vi "160041036.vi"() -> ()   [LabVIEW 2018]
panel:
  out "CAR":bool
  out "Boolean 19":bool
  out "Boolean 18":bool
  out "Boolean 17":bool
  out "Boolean 16":bool
  out "Boolean 15":bool
  out "Boolean 14":bool
  out "?":bool
  out "?":bool
  out "Boolean 13":bool
  out "Boolean 12":bool
  out "?":bool
  out "car 4":bool
  out "car 3":bool
  out "car2":bool
  out "1":bool
  out "2":bool
  in  "Boolean 11":bool
  in  "Boolean 10":bool
  in  "Boolean 9":bool
  in  "Boolean 8":bool
  in  "Boolean 7":bool
  in  "Boolean 6":bool
  in  "Boolean 5":bool
  in  "Boolean 4":bool
  in  "Boolean 3":bool
  in  "Boolean 2":bool
  in  "Boolean":bool
  # "R.R. MALL PARKING"
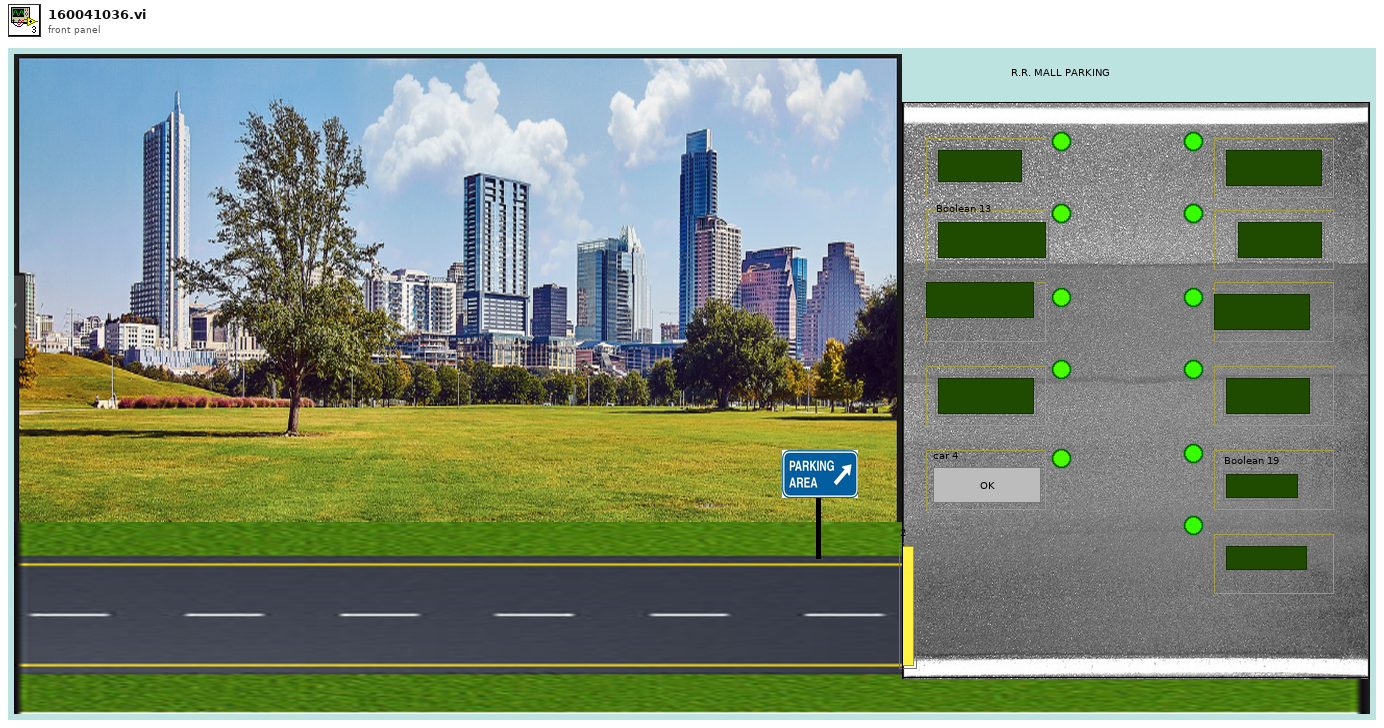
[diagram p1: front panel]
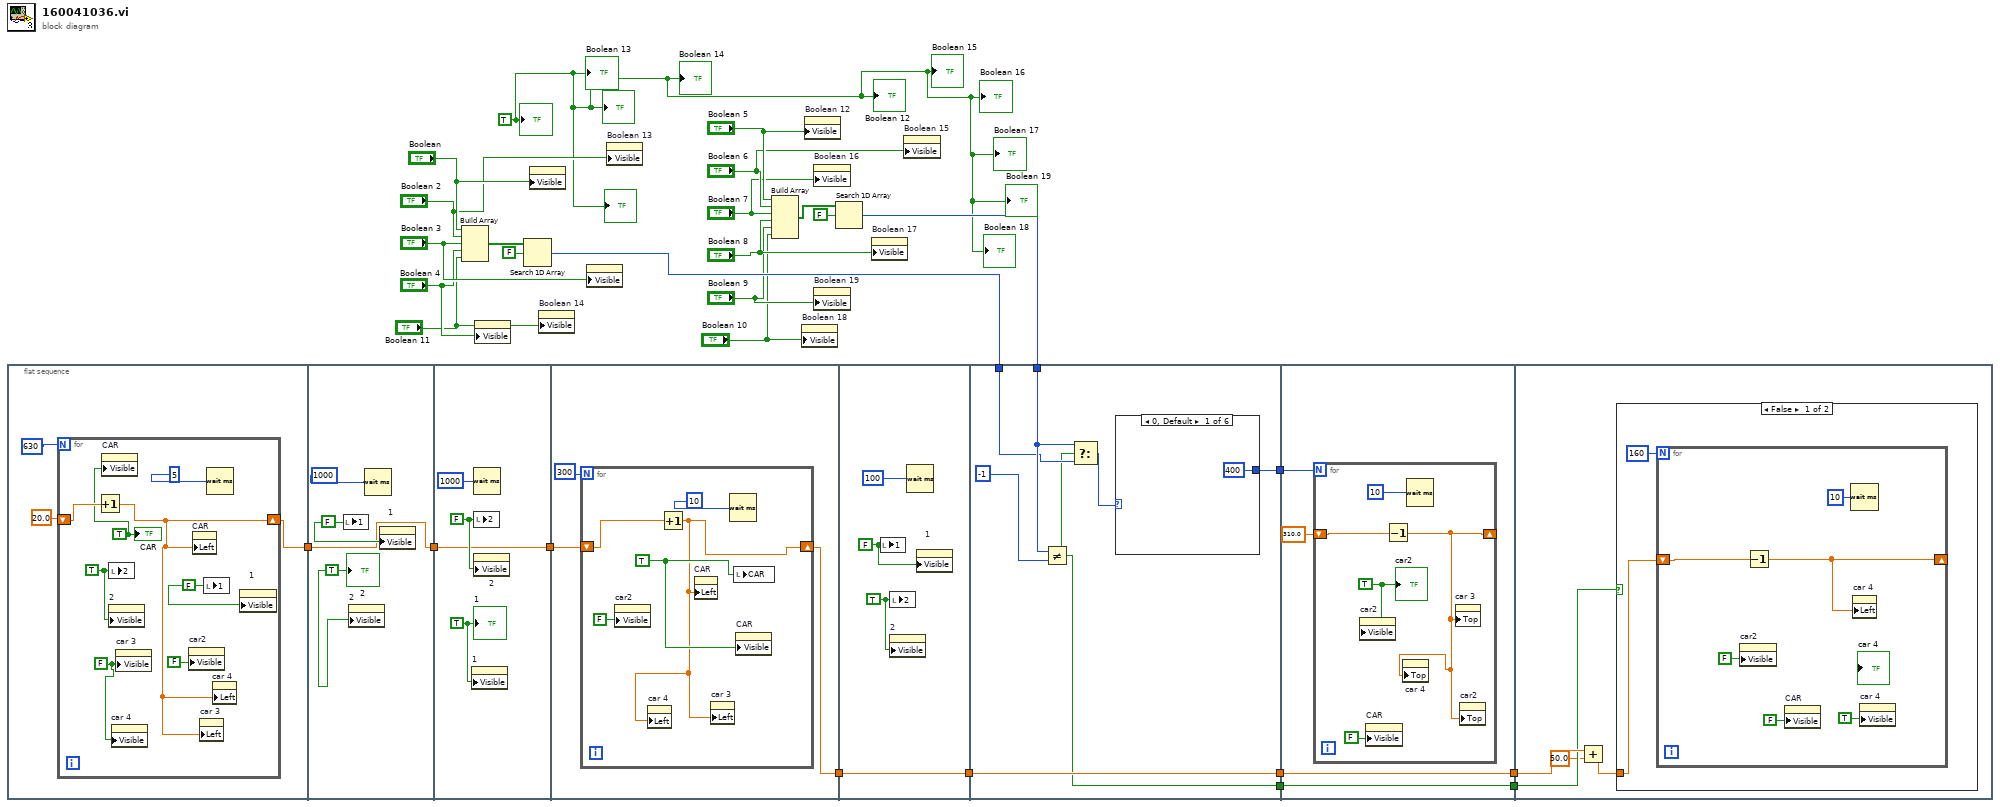
[diagram p0: block diagram]
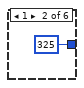
[diagram p2: hidden frame]
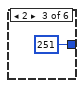
[diagram p3: hidden frame]
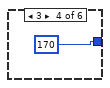
[diagram p4: hidden frame]
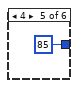
[diagram p5: hidden frame]
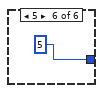
[diagram p6: hidden frame]
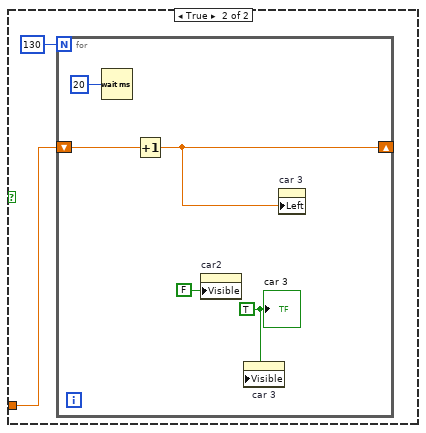
[diagram p7: hidden frame]
diagram:
  w3 = TRUE
  n1 = flat-sequence {
    tunnel: [w30] -> w24
    tunnel: w24 -> [w40]
    tunnel: [w40] -> w23
    tunnel: w23 -> [w44]
    tunnel: [w44] -> w22
    tunnel: w22 -> [w49]
    tunnel: [w48] -> w18
    tunnel: w18 -> [w56]
    tunnel: [w56] -> w17
    tunnel: w21 -> [w66]
    tunnel: [w64] -> w20
    tunnel: w19 -> [w62]
    tunnel: w17 -> [w61]
    tunnel: [w61] -> w16
    tunnel: [w60] -> w13
    tunnel: w20 -> [w75]
    tunnel: w16 -> [w74]
    tunnel: [w74] -> w15
    tunnel: [w73] -> w14
    tunnel: w13 -> [w73]
    tunnel: w15 -> [w85]
    tunnel: w14 -> [w84]
    frame #0 {
      n2 = for {
        N: 630 -> [_]
        shift-right: [w32] -> w30
        shift-left: 20.0 -> [w39]
        w33 = FALSE ("Visible")
        w36 = TRUE ("2")
        w37 = FALSE ("1")
        w35 = TRUE
        n3 = Increment(x=w39) -> (x+1=w32:dbl)
        n4 = property on="CAR" class="Bool (strict)"("Visible"=w35) -> ()  [unwired: 2 in, 2 out]
        n5 = local write "2"(w36) -> ()
        n6 = property on="2" class="Bool (strict)"("Visible"=w36) -> ()  [unwired: 2 in, 2 out]
        n7 = property on="car 4" class="Bool"("Visible"=w33) -> ()  [unwired: 2 in, 2 out]
        n8 = property on="car 3" class="Bool"("Visible"=w33) -> ()  [unwired: 2 in, 2 out]
        n9 = property on="car2" class="Bool"("Visible"=FALSE) -> ()  [unwired: 2 in, 2 out]
        n10 = property on="CAR" class="Bool (strict)"("Left"=w32) -> ()  [unwired: 2 in, 2 out]
        n11 = property on="car 3" class="Bool"("Left"=w32) -> ()  [unwired: 2 in, 2 out]
        n12 = local write "1"(w37) -> ()
        n13 = Wait (ms)(milliseconds to wait=u32 5 ("millisecond timer value")) -> ()  [unwired: 1 out]
        n14 = property on="car 4" class="Bool"("Left"=w32) -> ()  [unwired: 2 in, 2 out]
        n15 = property on="1" class="Bool (strict)"("Visible"=w37) -> ()  [unwired: 2 in, 2 out]
        "CAR" <- w35
      }
    }
    frame #1 {
      w41 = FALSE ("1")
      w42 = TRUE ("Boolean 12")
      n16 = local write "1"(w41) -> ()
      n17 = property on="2" class="Bool (strict)"("Visible"=w42) -> ()  [unwired: 2 in, 2 out]
      n18 = Wait (ms)(milliseconds to wait=u32 1000 ("millisecond timer value")) -> ()  [unwired: 1 out]
      n19 = property on="1" class="Bool (strict)"("Visible"=w41) -> ()  [unwired: 2 in, 2 out]
      "2" <- w42
    }
    frame #2 {
      w45 = FALSE ("2")
      w46 = TRUE ("1")
      n20 = property on="1" class="Bool (strict)"("Visible"=w46) -> ()  [unwired: 2 in, 2 out]
      n21 = Wait (ms)(milliseconds to wait=u32 1000 ("millisecond timer value")) -> ()  [unwired: 1 out]
      n22 = local write "2"(w45) -> ()
      n23 = property on="2" class="Bool (strict)"("Visible"=w45) -> ()  [unwired: 2 in, 2 out]
      "1" <- w46
    }
    frame #3 {
      n24 = for {
        N: 300 -> [_]
        shift-right: [w51] -> w48
        shift-left: w49 -> [w54]
        w53 = TRUE
        n25 = property on="car2" class="Bool"("Visible"=FALSE) -> ()  [unwired: 2 in, 2 out]
        n26 = Increment(x=w54) -> (x+1=w51:dbl)
        n27 = property on="car 4" class="Bool"("Left"=w51) -> ()  [unwired: 2 in, 2 out]
        n28 = property on="CAR" class="Bool (strict)"("Left"=w51) -> ()  [unwired: 2 in, 2 out]
        n29 = property on="car 3" class="Bool"("Left"=w51) -> ()  [unwired: 2 in, 2 out]
        n30 = Wait (ms)(milliseconds to wait=u32 10 ("millisecond timer value")) -> ()  [unwired: 1 out]
        n31 = local write "CAR"(w53) -> ()
        n32 = property on="CAR" class="Bool (strict)"("Visible"=w53) -> ()  [unwired: 2 in, 2 out]
      }
    }
    frame #4 {
      w58 = FALSE ("1")
      w59 = TRUE ("2")
      n33 = local write "1"(w58) -> ()
      n34 = local write "2"(w59) -> ()
      n35 = property on="2" class="Bool (strict)"("Visible"=w59) -> ()  [unwired: 2 in, 2 out]
      n36 = Wait (ms)(milliseconds to wait=u32 100 ("millisecond timer value")) -> ()  [unwired: 1 out]
      n37 = property on="1" class="Bool (strict)"("Visible"=w58) -> ()  [unwired: 2 in, 2 out]
    }
    frame #5 {
      n38 = Not Equal?(x=w66, y=-1) -> (x != y?=w60:bool)
      n39 = Select(t=w66, s=w60, f=w62) -> (s? t:f=w65:i32)
      n40 = case shown="0, Default" w65 {
        tunnel: [400 ("y") 325 ("y") 251 ("y") 170 ("y") 85 5] -> w64
        frame 0, Default {
        }
        frame 1 {
        }
        frame 2 {
        }
        frame 3 {
        }
        frame 4 {
        }
        frame 5 {
        }
      }
    }
    frame #6 {
      n41 = for {
        N: w75 -> [_]
        shift-right: [w77] -> _
        shift-left: 310.0 -> [w81]
        w79 = TRUE ("CAR")
        n42 = property on="car2" class="Bool"("Visible"=w79) -> ()  [unwired: 2 in, 2 out]
        n43 = property on="CAR" class="Bool (strict)"("Visible"=FALSE) -> ()  [unwired: 2 in, 2 out]
        n44 = Decrement(x=w81) -> (x-1=w77:dbl)
        n45 = property on="car 4" class="Bool"("Top"=w77) -> ()  [unwired: 2 in, 2 out]
        n46 = Wait (ms)(milliseconds to wait=u32 10 ("millisecond timer value")) -> ()  [unwired: 1 out]
        n47 = property on="car 3" class="Bool"("Top"=w77) -> ()  [unwired: 2 in, 2 out]
        n48 = property on="car2" class="Bool"("Top"=w77) -> ()  [unwired: 2 in, 2 out]
        "car2" <- w79
      }
    }
    frame #7 {
      n49 = Add(x=w85, y=50.0) -> (x+y=w83:dbl)
      n50 = case shown="False" w84 {
        tunnel: w83 -> [w87 w94]
        frame False {
          n51 = for {
            N: 160 -> [_]
            shift-right: [w92] -> _
            shift-left: w87 -> [w93]
            n52 = property on="car2" class="Bool"("Visible"=FALSE) -> ()  [unwired: 2 in, 2 out]
            n53 = Decrement(x=w93) -> (x-1=w92:dbl)
            n54 = property on="CAR" class="Bool (strict)"("Visible"=FALSE) -> ()  [unwired: 2 in, 2 out]
            n55 = Wait (ms)(milliseconds to wait=u32 10) -> ()  [unwired: 1 out]
            n56 = property on="car 4" class="Bool"("Left"=w92) -> ()  [unwired: 2 in, 2 out]
            n57 = property on="car 4" class="Bool"("Visible"=TRUE) -> ()  [unwired: 2 in, 2 out]
          }
        }
        frame True {
          n58 = for {
            N: 130 -> [_]
            shift-right: [w97] -> _
            shift-left: w94 -> [w100]
            w96 = TRUE ("car 3")
            n59 = Wait (ms)(milliseconds to wait=u32 20 ("millisecond timer value")) -> ()  [unwired: 1 out]
            n60 = Increment(x=w100) -> (x+1=w97:dbl)
            n61 = property on="car2" class="Bool"("Visible"=FALSE) -> ()  [unwired: 2 in, 2 out]
            n62 = property on="car 3" class="Bool"("Visible"=w96) -> ()  [unwired: 2 in, 2 out]
            n63 = property on="car 3" class="Bool"("Left"=w97) -> ()  [unwired: 2 in, 2 out]
            "car 3" <- w96
          }
        }
      }
    }
  }
  n64 = Build Array("Boolean", "Boolean 2", "Boolean 3", "Boolean 4", "Boolean 11") -> (w28:bool[])
  n65 = property class="Bool (strict)"("Visible"="Boolean 4") -> ()  [unwired: 2 in, 2 out]
  n66 = Search 1D Array(1D array=w28, element=FALSE) -> (index of element=w19:i32)  [unwired: 1 in]
  n67 = property class="Bool (strict)"("Visible"="Boolean") -> ()  [unwired: 2 in, 2 out]
  n68 = property on="Boolean 14" class="Bool (strict)"("Visible"="Boolean 11") -> ()  [unwired: 2 in, 2 out]
  n69 = property class="Bool (strict)"("Visible"="Boolean 3") -> ()  [unwired: 2 in, 2 out]
  n70 = property on="Boolean 13" class="Bool (strict)"("Visible"="Boolean 2") -> ()  [unwired: 2 in, 2 out]
  n71 = Build Array("Boolean 5", "Boolean 6", "Boolean 7", "Boolean 8", "Boolean 9", "Boolean 10") -> (w25:bool[])
  n72 = property on="Boolean 18" class="Bool (strict)"("Visible"="Boolean 10") -> ()  [unwired: 2 in, 2 out]
  n73 = property on="Boolean 12" class="Bool (strict)"("Visible"="Boolean 5") -> ()  [unwired: 2 in, 2 out]
  n74 = property on="Boolean 16" class="Bool (strict)"("Visible"="Boolean 7") -> ()  [unwired: 2 in, 2 out]
  n75 = property on="Boolean 19" class="Bool (strict)"("Visible"="Boolean 9") -> ()  [unwired: 2 in, 2 out]
  n76 = Search 1D Array(1D array=w25, element=FALSE) -> (index of element=w21:i32)  [unwired: 1 in]
  n77 = property on="Boolean 17" class="Bool (strict)"("Visible"="Boolean 8") -> ()  [unwired: 2 in, 2 out]
  n78 = property on="Boolean 15" class="Bool (strict)"("Visible"="Boolean 6") -> ()  [unwired: 2 in, 2 out]
  "?" <- w3
  "Boolean 13" <- w3
  "?" <- w3
  "?" <- w3
  "Boolean 14" <- w3
  "Boolean 12" <- w3
  "Boolean 15" <- w3
  "Boolean 16" <- w3
  "Boolean 17" <- w3
  "Boolean 18" <- w3
  "Boolean 19" <- w3
